vi "GetTimeStr.vi"(4 "时间标识":timestamp) -> (1 "字符串":string)   [LabVIEW 2018]
doc: "获取短时间格式的字符串，未输入时间标识时，默认返回当前时间的字符串"
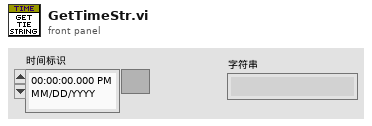
[diagram p1: front panel]
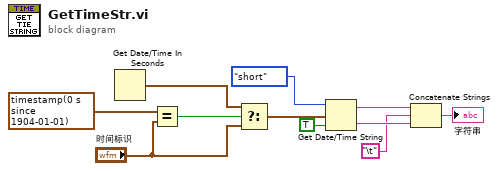
[diagram p0: block diagram]
diagram:
  n1 = Get Date/Time In Seconds() -> (seconds since 1Jan1904=w4:timestamp)
  n2 = Equal?(x=timestamp(0 s since 1904-01-01), y="时间标识") -> (x = y?=w5:bool)
  n3 = Select(t=w4, s=w5, f="时间标识") -> (s? t:f=w2:timestamp)
  n4 = Get Date/Time String(date format (0)=enum16{"short", "long", "abbreviated"}."short" ("日期格式(0)"), seconds (now)=w2, want seconds? (F)=TRUE ("需要秒？(F)")) -> (date string=w11:string, time string=w10:string)
  n5 = Concatenate Strings(w11, "\t", w10) -> (→"字符串":string)
